vi "Logging Message Loop.vi"(8 "error in (no error)":errorcluster, 11 "Message Queues":T1) -> (0 "error out":errorcluster)   [LabVIEW 2018, in "Logging.lvlib"]
doc: "The message loop subVI to handle messages pertaining to logging data."
uses:
  Logging.lvlib
  Support/Message Queue/All Message Queues.ctl
  Support/Message Queue/Message Cluster.ctl
  Controls/Data Queue.ctl
  library/Datalogger LLB/Data Record Control.ctl
  Controls/Data Notifier.ctl
  Logging Configuration.ctl
  Logging State.ctl
  <vilib>/Utility/error.llb/Error Cluster From Error Code.vi
  <vilib>/ErrorRing/Error Ring.xnode
  support/Message Queue/Message Queue.lvlib
  library/Datalogger LLB/Datalogger.lvclass
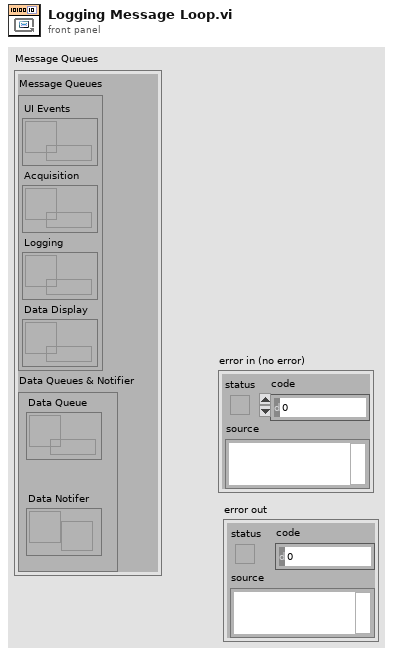
[diagram p1: front panel]
types:
  T1 = typedef "Message Queue.lvlib/All Message Queues.ctl" = cluster{"Message Queues":cluster{"UI Events":refnum<queue>, "Acquisition":refnum<queue>, "Logging":refnum<queue>, "Data Display":refnum<queue>}, "Data Queues & Notifier":cluster{"Data Queue":T2, "Data Notifer":T3}}
  T2 = typedef "Data Queue.ctl" = refnum<queue>
  T3 = typedef "Data Notifier.ctl" = refnum<notifier>
  T4 = typedef "Logging.lvlib/Logging Configuration.ctl" = cluster{"Log File Base Path":path, "TDMS File Reference":refnum<k34>}
  T5 = typedef "Logging.lvlib/Logging State.ctl" = enum16{"Idle", "Logging"}
  T6 = enum16{"open", "open or create", "create or replace", "create", "open (read-only)"}
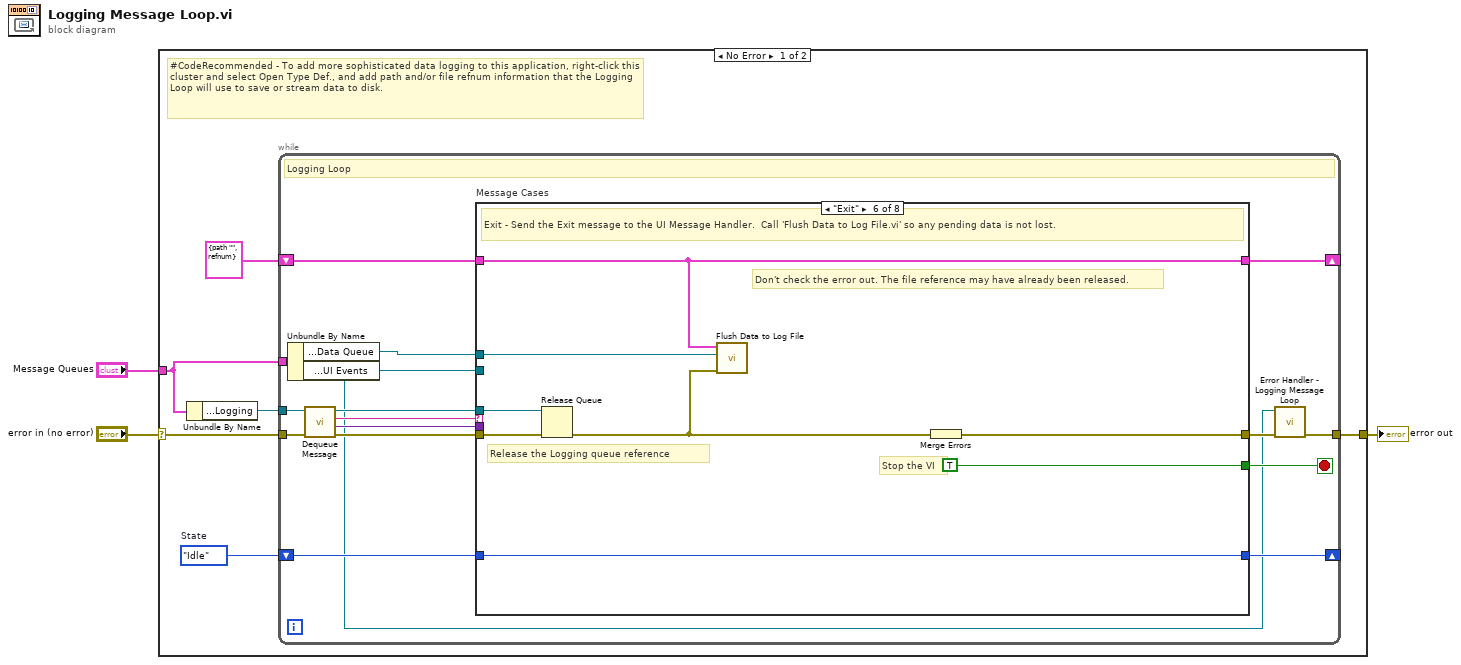
[diagram p0: block diagram]
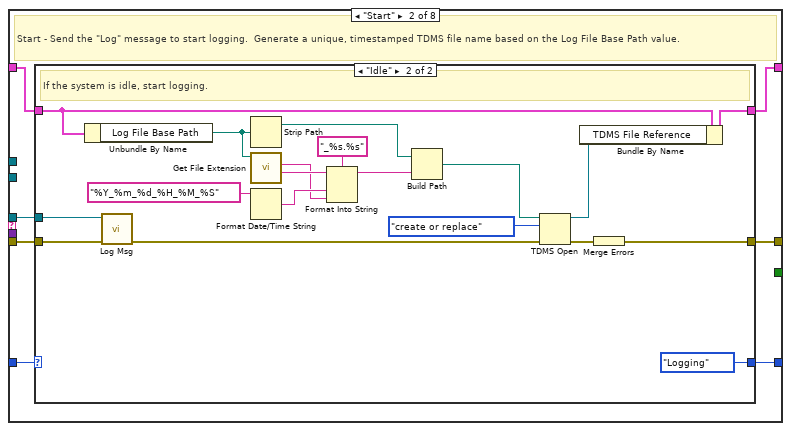
[diagram p3: hidden frame]
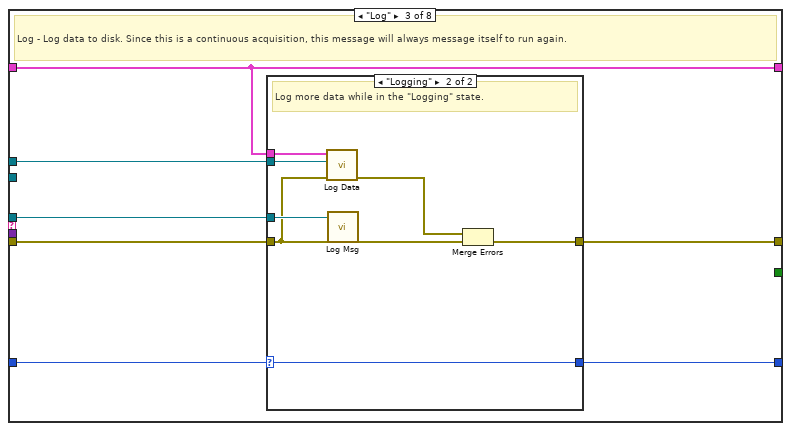
[diagram p5: hidden frame]
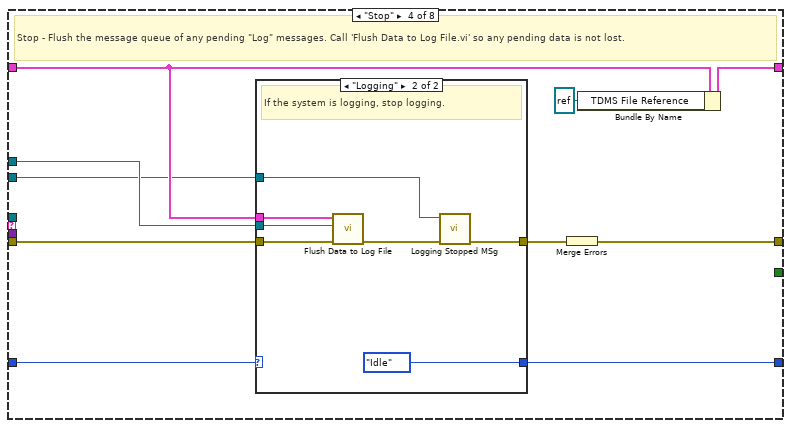
[diagram p7: hidden frame]
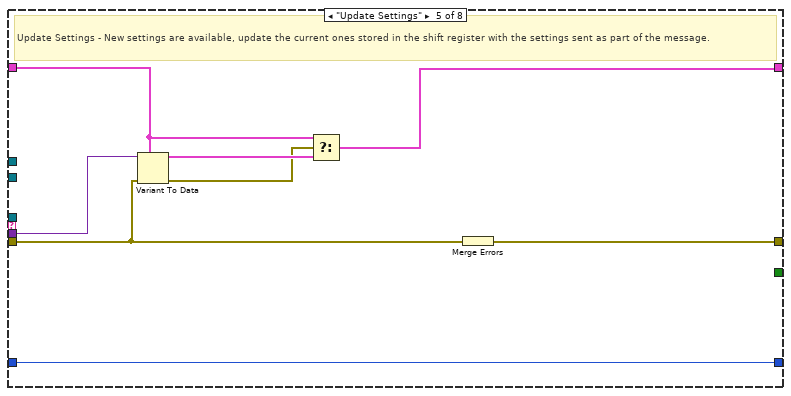
[diagram p9: hidden frame]
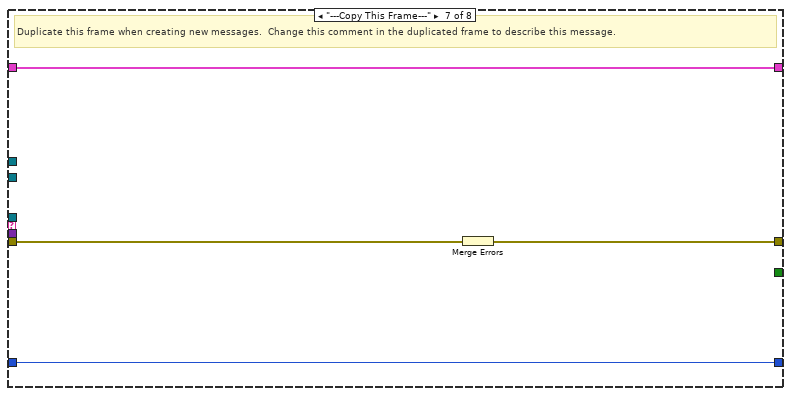
[diagram p10: hidden frame]
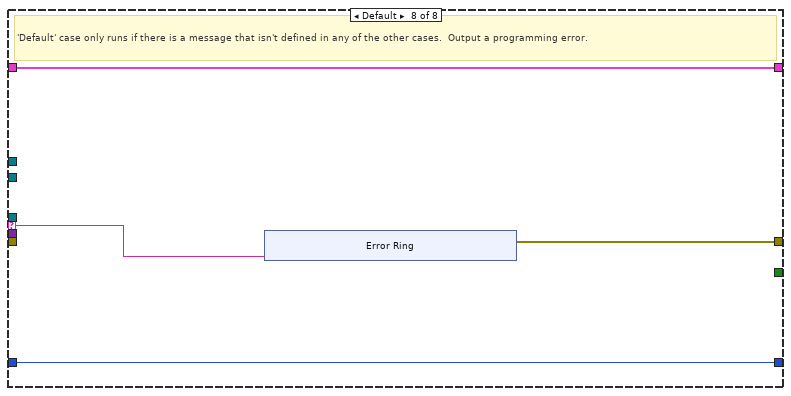
[diagram p11: hidden frame]
diagram:
  n1 = case shown="No Error" "error in (no error)" {
    selector: "error in (no error)" -> [w6 w125]
    tunnel: "Message Queues" -> [w4 _]
    tunnel: [w8 w125] -> w2
    frame No Error {
      w5 = Logging_State."Idle"  # State
      # "#CodeRecommended - To add more sophisticated data logging to this application, right-click this cluster and select Open Type Def., and add path and/or file refnum information that the Logging Loop will use to save or stream data to disk."
      n2 = Unbundle By Name(w4) -> ("Message Queues.Logging"=w9:refnum<queue>)
      n3 = while {
        tunnel: w9 -> [w17]
        shift-right: [w24] -> _
        shift-left: T4 {"Log File Base Path"=path "", "TDMS File Reference"=refnum} ("Logging Configuration") -> [w25]
        shift-right: [w15] -> _
        shift-left: w5 -> [w16]
        tunnel: w6 -> [w22]
        tunnel: [w14] -> w8
        tunnel: w4 -> [w12]
        stop <- w23 stop-if-true
        # "Logging Loop"
        n4 = Unbundle By Name(w12) -> ("Data Queues & Notifier.Data Queue"=w11:T2, "Message Queues.UI Events"=w10:refnum<queue>)
        n5 = call "Dequeue Message.vi"("error in (no error)"=w22, "Message Queue"=w17) -> ("error out"=w21:errorcluster, "Message Data"=w19:variant, "Message"=w20:string, "dup Message Queue"=w18:refnum<queue>)  [unwired: 6 in]
        n6 = case "Message Cases" shown="\"Exit\"" w20 {
          selector: w20 -> [_ _ _ _ _ _ _ w114]
          tunnel: w18 -> [_ w34 w63 _ _ w106 _ _]
          tunnel: w21 -> [w27 w33 w61 w78 w95 w107 w113 _]
          tunnel: [w27 w35 w64 w84 w101 w108 w111 w115] -> w13
          tunnel: w25 -> [w28 w32 w60 w79 w99 w104 w112 w117]
          tunnel: [w28 w31 w60 w82 w96 w104 w112 w117] -> w24
          tunnel: [_ _ _ _ _ TRUE _ _] -> w23
          tunnel: w19 -> [_ _ _ _ w100 _ _ _]
          tunnel: w10 -> [_ _ _ w75 _ _ _ _]
          tunnel: w11 -> [_ _ w62 w80 _ w103 _ _]
          tunnel: w16 -> [w26 w30 w59 w77 w94 w102 w110 w116]
          tunnel: [w26 w29 w58 w76 w94 w102 w110 w116] -> w15
          frame "Initialize" {
            # "Initialize - gets called when first launched. Currently a no-op."
          }
          frame "Start" {
            # "Start - Send the \"Log\" message to start logging.  Generate a unique, timestamped TDMS file name based on the Log File Base Path value."
            n7 = case shown="\"Idle\"" w30 {
              selector: w30 -> [w37 _]
              tunnel: [w36 w42] -> w35
              tunnel: w34 -> [_ w40]
              tunnel: w33 -> [w36 w41]
              tunnel: w32 -> [w38 w43]
              tunnel: [w38 w45] -> w31
              tunnel: [w37 Logging_State."Logging" ("State")] -> w29
              frame "Logging" {
                # "The system is already logging. Ignore the \"Start\" message."
              }
              frame "Idle" {
                # "If the system is idle, start logging."
                n8 = Unbundle By Name(w43) -> ("Log File Base Path"=w57:path)
                n9 = call "Log Msg.vi"("error in (no error)"=w41, "Queue in"=w40) -> ("error out"=w39:errorcluster)  [unwired: 9 in]
                n10 = Strip Path(path=w57) -> (stripped path=w54:path)  [unwired: 1 out]
                n11 = call <vilib>:"Get File Extension.vi"("file"=w57) -> ("filename without extension"=w55:string, "lowercase file extension"=w51:string)  [unwired: 6 in, 3 out]
                n12 = Format Date/Time String(time format string (%c)="%Y_%m_%d_%H_%M_%S") -> (date/time string=w52:string)  [unwired: 2 in]
                n13 = Format Into String(format string="_%s.%s", initial string=w55, w52, w51) -> (resulting string=w50:string)  [unwired: 1 in, 1 out]
                n14 = Build Path(base path=w54, name or relative path=w50) -> (appended path=w49:path)
                n15 = TDMS Open(8:w39, 10:T6."create or replace" ("operation (0:open)"), 11:w49) -> (0:w48:errorcluster, 3:w46:refnum<k34>)  [unwired: 4 in]
                n16 = Bundle By Name(cluster=w43, "TDMS File Reference"=w46) -> (w45:T4)
                n17 = Merge Errors(w48) -> (w42:errorcluster)
              }
            }
          }
          frame "Log" {
            # "Log - Log data to disk. Since this is a continuous acquisition, this message will always message itself to run again."
            n18 = case shown="\"Logging\"" w59 {
              selector: w59 -> [w66 w68]
              tunnel: [w65 w74] -> w64
              tunnel: w63 -> [_ w72]
              tunnel: w62 -> [_ w71]
              tunnel: w61 -> [w65 w67]
              tunnel: w60 -> [_ w69]
              tunnel: [w66 w68] -> w58
              frame "Idle" {
                # "Ignore \"Log\" messages when the logging is idle."
              }
              frame "Logging" {
                # "Log more data while in the \"Logging\" state."
                n19 = call "Log Data.vi"("error in (no error)"=w67, "Data Queue"=w71, "Logging Configuration"=w69) -> ("error out"=w70:errorcluster)  [unwired: 8 in]
                n20 = call "Log Msg.vi"("error in (no error)"=w67, "Queue in"=w72) -> ("error out"=w73:errorcluster)  [unwired: 9 in]
                n21 = Merge Errors(w70, w73) -> (w74:errorcluster)
              }
            }
          }
          frame "Stop" {
            # "Stop - Flush the message queue of any pending \"Log\" messages. Call 'Flush Data to Log File.vi' so any pending data is not lost."
            n22 = case shown="\"Logging\"" w77 {
              selector: w77 -> [w85 _]
              tunnel: [w86 w88] -> w83
              tunnel: w80 -> [_ w92]
              tunnel: w79 -> [_ w91]
              tunnel: w78 -> [w86 w90]
              tunnel: [w85 Logging_State."Idle" ("State")] -> w76
              tunnel: w75 -> [_ w87]
              frame "Idle" {
                # "The system is already idle. Ignore the \"Stop\" message."
              }
              frame "Logging" {
                # "If the system is logging, stop logging."
                n23 = call "Flush Data to Log File.vi"("error in (no error)"=w90, "Data Queue"=w92, "Logging Configuration"=w91) -> ("error out"=w93:errorcluster)  [unwired: 8 in]
                n24 = call "Logging Stopped MSg.vi"("error in (no error)"=w93, "Queue in"=w87) -> ("error out"=w88:errorcluster)  [unwired: 9 in]
              }
            }
            n25 = Merge Errors(w83) -> (w84:errorcluster)
            n26 = Bundle By Name(cluster=w79, "TDMS File Reference"=refnum<k34> refnum) -> (w82:T4)
          }
          frame "Update Settings" {
            # "Update Settings - New settings are available, update the current ones stored in the shift register with the settings sent as part of the message."
            n27 = Variant To Data(error in=w95, type=w99, Variant=w100) -> (data=w98:T4, error out=w97:errorcluster)
            n28 = Select(t=w99, s=w97, f=w98) -> (s? t:f=w96:T4)
            n29 = Merge Errors(w95) -> (w101:errorcluster)
          }
          frame "Exit" {
            # "Don't check the error out. The file reference may have already been released."
            # "Release the Logging queue reference"
            # "Stop the VI"
            # "Exit - Send the Exit message to the UI Message Handler.  Call 'Flush Data to Log File.vi' so any pending data is not lost."
            n30 = Release Queue(queue=w106, error in (no error)=w107) -> (error out=w105:errorcluster)  [unwired: 1 in, 2 out]
            n31 = call "Flush Data to Log File.vi"("error in (no error)"=w105, "Data Queue"=w103, "Logging Configuration"=w104) -> ()  [unwired: 8 in, 1 out]
            n32 = Merge Errors(w105) -> (w108:errorcluster)
          }
          frame "---Copy This Frame---" {
            # "Duplicate this frame when creating new messages.  Change this comment in the duplicated frame to describe this message."
            n33 = Merge Errors(w113) -> (w111:errorcluster)
          }
          frame Default {
            # "'Default' case only runs if there is a message that isn't defined in any of the other cases.  Output a programming error."
            n34 = xnode "Error Ring"("parameter 0"=w114) -> ("error out"=w115:errorcluster)
          }
        }
        n35 = call "Error Handler - Logging Message Loop.vi"("error in (no error)"=w13, "Message Queue"=w10) -> ("dup error in"=w14:errorcluster)  [unwired: 8 in, 1 out]
      }
    }
    frame Error {
    }
  }
  "error out" <- w2
